vi "Load AI Driver.vi"(8 "error in (no error)":errorcluster, 9 "Config Path":path, 10 "Section":string, 11 "Test Station SIM AI Factory in":refnum<class "Test Station SIM AI Factory.lvclass">) -> (0 "error out":errorcluster, 2 "AI Driver.lvclass":refnum<class "AI Driver.lvclass">)   [LabVIEW 2022 SP3, in "Test Station SIM AI Factory.lvclass"]
uses:
  Test Station SIM AI Factory.lvclass
  AI Driver/AI Driver.lvclass
  Test Station SIM AI Factory.lvclass/Test Station SIM AI Factory.ctl
  Test Station SIM AI Driver/Test Station SIM AI Driver.lvclass
  C:/XY Stage/IO Monitor/SIM AI Driver/SIM AI Driver.lvclass
  C:/XY Stage/IO Monitor/AI Driver/AI Driver.lvclass
  C:/XY Stage/IO Monitor/Test Station SIM AI Driver/Test Station SIM AI Driver.lvclass
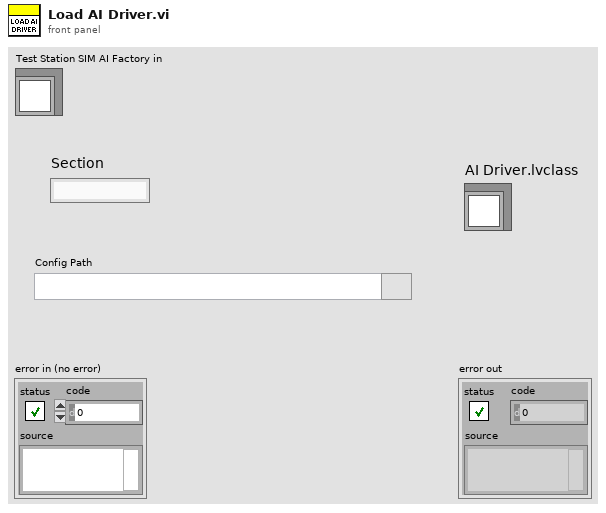
[diagram p1: front panel]
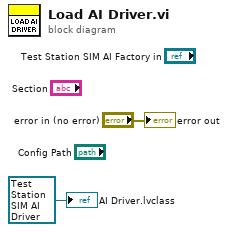
[diagram p0: block diagram]
diagram:
  "error out" <- "error in (no error)"
  "AI Driver.lvclass" <- refnum<class "Test Station SIM AI Driver.lvclass"> refnum ("Test Station SIM AI Driver.lvclass")
